vi "read-multiple-registers-rack.vi"(8 "error in":errorcluster, 9 "regs":u16[](array[numeric]), 10 "number of input registers":u16, 11 "TCP master in":refnum<class "Modbus Master.lvclass">) -> (0 "error out":errorcluster, 2 "Rack Cluster":T1, 3 "Modbus master out":refnum<class "Modbus Master.lvclass">)   [LabVIEW 2021]
uses:
  <vilib>/Modbus/master/Modbus Master.lvclass
  General Purpose/BMS.ctl
panel:
  in  "id":u16
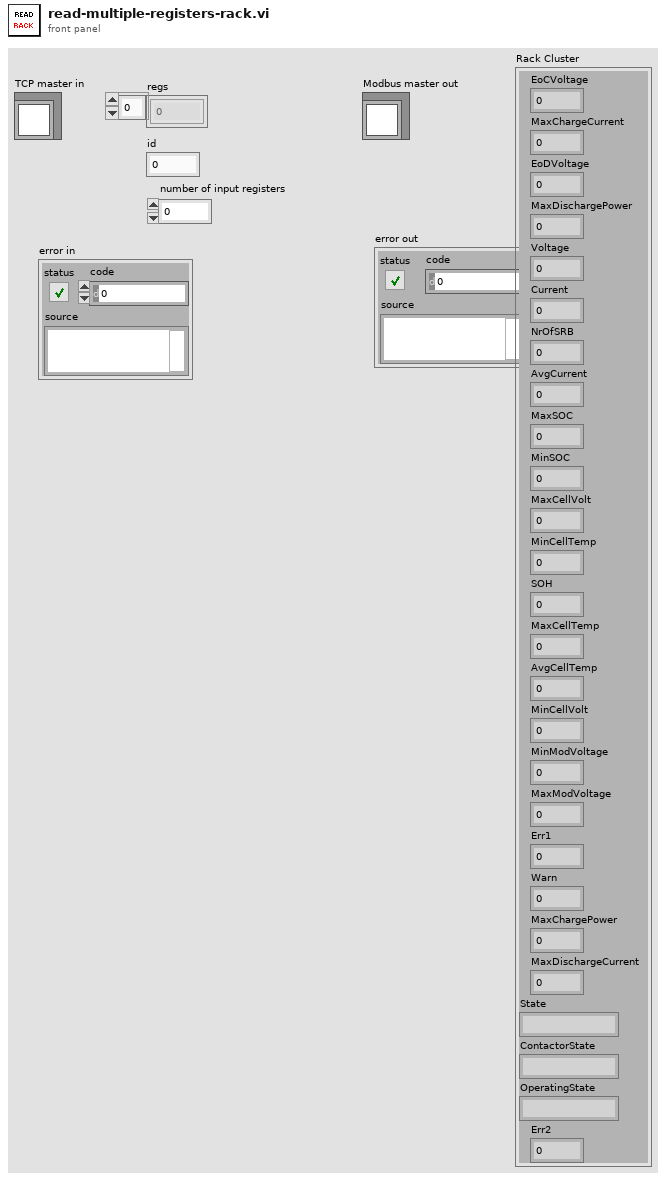
[diagram p1: front panel]
types:
  T1 = cluster{"EoCVoltage":dbl, "MaxChargeCurrent":dbl, "EoDVoltage":dbl, "MaxDischargePower":dbl, "Voltage":dbl, "Current":dbl, "NrOfSRB":u16, "AvgCurrent":dbl, "MaxSOC":u16, "MinSOC":u16, "MaxCellVolt":dbl, "MinCellTemp":dbl, "SOH":u16, "MaxCellTemp":dbl, "AvgCellTemp":dbl, "MinCellVolt":dbl, "MinModVoltage":dbl, "MaxModVoltage":dbl, "Err1":u16, "Warn":u16, "MaxChargePower":dbl, "MaxDischargeCurrent":dbl, "State":string, "ContactorState":string, "OperatingState":string, "Err2":u16}
  T2 = typedef "BMS.ctl" = cluster{"rack":cluster{"EoCVoltage":dbl, "MaxChargeCurrent":dbl, "EoDVoltage":dbl, "MaxDischargePower":dbl, "Voltage":dbl, "Current":dbl, "NrOfSRB":u16, "AvgCurrent":dbl, "MaxSOC":u16, "MinSOC":u16, "MaxCellVolt":dbl, "MinCellTemp":dbl, "SOH":u16, "MaxCellTemp":dbl, "AvgCellTemp":dbl, "MinCellVolt":dbl, "MinModVoltage":dbl, "MaxModVoltage":dbl, "Err1":u16, "Warn":u16, "MaxChargePower":dbl, "MaxDischargeCurrent":dbl, "State":string, "ContactorState":string, "OperatingState":string, "Err2":u16}[], "modules":cluster{"Voltage":dbl, "MaxCellTemp":dbl, "AirTempIn":dbl, "MinCellVoltage":u16, "AirTempOut":dbl, "MinSOC":u16, "MaxCellVoltage":u16, "Warn":u16, "SOH":u16, "MinCellTemp":dbl, "Err":u16, "Max SOC":u16}[]}
  T3 = cluster{"EoCVoltage":dbl, "MaxChargeCurrent":dbl, "EoDVoltage":dbl, "MaxDischargePower":dbl, "Voltage":dbl, "Current":dbl, "NrOfSRB":u16, "AvgCurrent":dbl, "MaxSOC":u16, "MinSOC":u16, "MaxCellVolt":dbl, "MinCellTemp":dbl, "SOH":u16, "MaxCellTemp":dbl, "AvgCellTemp":dbl, "MinCellVolt":dbl, "MinModVoltage":dbl, "MaxModVoltage":dbl, "Err1":u16, "Warn":u16, "MaxChargePower":dbl, "MaxDischargeCurrent":dbl, "State":string, "ContactorState":string, "OperatingState":string, "Err2":u16}[]
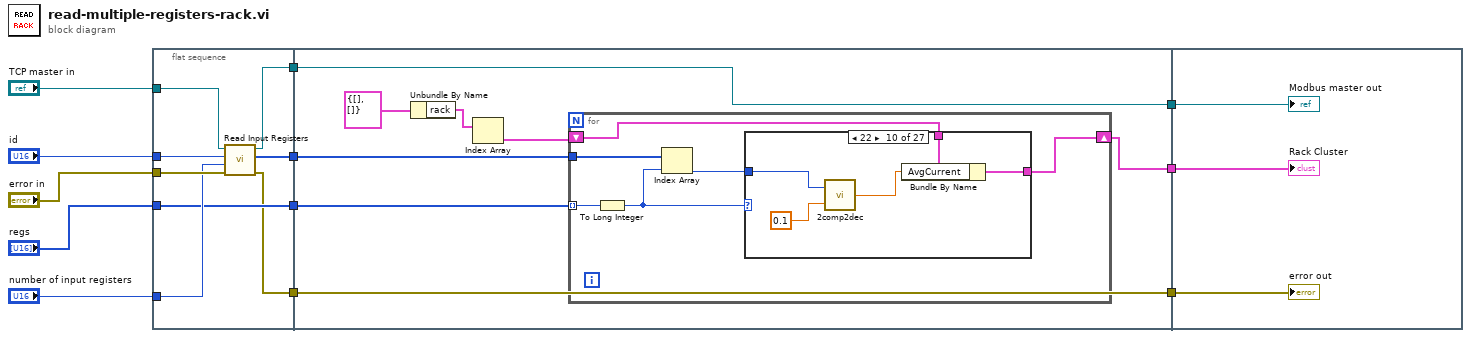
[diagram p0: block diagram]
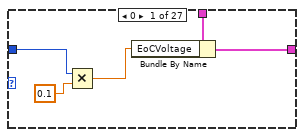
[diagram p2: hidden frame]
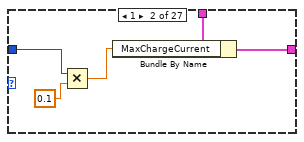
[diagram p3: hidden frame]
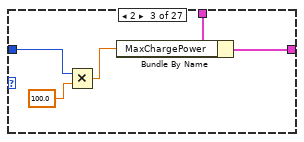
[diagram p4: hidden frame]
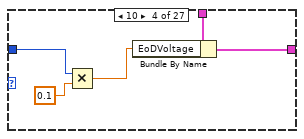
[diagram p5: hidden frame]
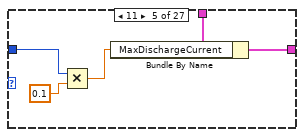
[diagram p6: hidden frame]
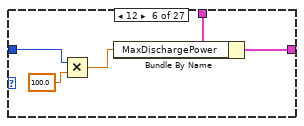
[diagram p7: hidden frame]
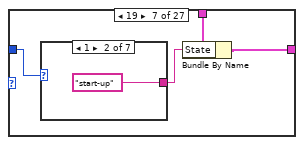
[diagram p8: hidden frame]
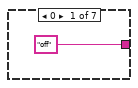
[diagram p9: hidden frame]
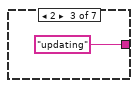
[diagram p10: hidden frame]
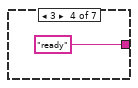
[diagram p11: hidden frame]
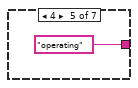
[diagram p12: hidden frame]
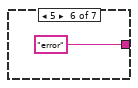
[diagram p13: hidden frame]
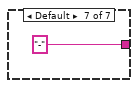
[diagram p14: hidden frame]
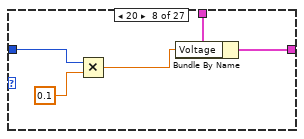
[diagram p15: hidden frame]
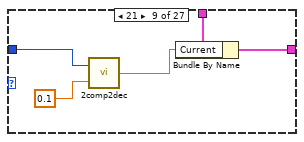
[diagram p16: hidden frame]
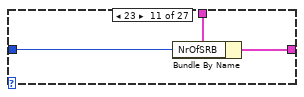
[diagram p17: hidden frame]
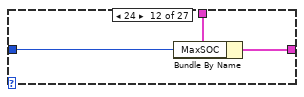
[diagram p18: hidden frame]
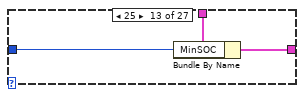
[diagram p19: hidden frame]
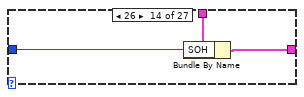
[diagram p20: hidden frame]
diagram:
  n1 = flat-sequence {
    tunnel: "TCP master in" -> [w20]
    tunnel: "id" -> [w19]
    tunnel: "error in" -> [w18]
    tunnel: "number of input registers" -> [w17]
    tunnel: [w16] -> w8
    tunnel: "regs" -> [w16]
    tunnel: [w15] -> w6
    tunnel: [w14] -> w3
    tunnel: [w13] -> w2
    tunnel: w8 -> [w28]
    tunnel: w6 -> [w27]
    tunnel: [w23] -> w5
    tunnel: [w22] -> w4
    tunnel: w3 -> [w22]
    tunnel: w2 -> [w21]
    tunnel: [w21] -> w1
    tunnel: w5 -> [w162]
    tunnel: w4 -> [w164]
    tunnel: w1 -> [w163]
    frame #0 {
      n2 = call-dynamic "Read Input Registers.vi"("error in (no error)"=w18, "number of input registers"=w17, "starting address"=w19, "Modbus master in"=w20) -> ("error out"=w13:errorcluster, "register values"=w15:u16[], "Modbus master out"=w14:refnum<class "Modbus Master.lvclass">)  [unwired: 5 in]
    }
    frame #1 {
      n3 = Unbundle By Name(T2 {"rack"=[], "modules"=[]} ("BMS")) -> ("rack"=w25:T3)
      n4 = Index Array(array=w25) -> (element=w24:T1)  [unwired: 1 in]
      n5 = for {
        tunnel: w28 -> [w34] mode=indexing
        tunnel: w27 -> [w33]
        shift-right: [w29] -> w23
        shift-left: w24 -> [w30]
        n6 = To Long Integer(number=w34) -> (32bit integer=w31:i32)
        n7 = Index Array(array=w33, index=w31) -> (element=w32:u16)
        n8 = case shown="22" w31 {
          tunnel: w32 -> [w37 w42 w46 w52 w57 w61 w66 w77 w83 w87 w91 w94 w97 w100 w104 w109 w117 w122 w127 w131 w134 w139 w145 w152 w155 w158 _]
          tunnel: w30 -> [w39 w44 w49 w54 w59 w64 w68 w80 w85 w90 w93 w96 w99 w102 w107 w111 w120 w125 w129 w133 w138 w143 w147 w154 w157 w160 w161]
          tunnel: [w38 w43 w48 w53 w58 w63 w67 w79 w84 w89 w92 w95 w98 w101 w106 w110 w119 w124 w128 w132 w137 w142 w146 w153 w156 w159 w161] -> w29
          frame 0 {
            n9 = Multiply(x=w37, y=0.1) -> (x*y=w36:dbl)
            n10 = Bundle By Name(cluster=w39, "EoCVoltage"=w36) -> (w38:T1)
          }
          frame 1 {
            n11 = Multiply(x=w42, y=0.1) -> (x*y=w40:dbl)
            n12 = Bundle By Name(cluster=w44, "MaxChargeCurrent"=w40) -> (w43:T1)
          }
          frame 2 {
            n13 = Multiply(x=w46, y=100.0) -> (x*y=w45:dbl)
            n14 = Bundle By Name(cluster=w49, "MaxChargePower"=w45) -> (w48:T1)
          }
          frame 10 {
            n15 = Multiply(x=w52, y=0.1 ("x")) -> (x*y=w50:dbl)
            n16 = Bundle By Name(cluster=w54, "EoDVoltage"=w50) -> (w53:T1)
          }
          frame 11 {
            n17 = Multiply(x=w57, y=0.1) -> (x*y=w55:dbl)
            n18 = Bundle By Name(cluster=w59, "MaxDischargeCurrent"=w55) -> (w58:T1)
          }
          frame 12 {
            n19 = Multiply(x=w61, y=100.0) -> (x*y=w60:dbl)
            n20 = Bundle By Name(cluster=w64, "MaxDischargePower"=w60) -> (w63:T1)
          }
          frame 19 {
            n21 = case shown="1" w66 {
              tunnel: ["off" "start-up" "updating" "ready" "operating" "error" "-"] -> w65
              frame 0 {
              }
              frame 1 {
              }
              frame 2 {
              }
              frame 3 {
              }
              frame 4 {
              }
              frame 5 {
              }
              frame Default {
              }
            }
            n22 = Bundle By Name(cluster=w68, "State"=w65) -> (w67:T1)
          }
          frame 20 {
            n23 = Multiply(x=w77, y=0.1) -> (x*y=w76:dbl)
            n24 = Bundle By Name(cluster=w80, "Voltage"=w76) -> (w79:T1)
          }
          frame 21 {
            n25 = call "2comp2dec.vi"("factor"=0.1, "two' complement"=w83) -> ("decimal"=w82:dbl)  [unwired: 1 in]
            n26 = Bundle By Name(cluster=w85, "Current"=w82) -> (w84:T1)
          }
          frame 22 {
            n27 = call "2comp2dec.vi"("factor"=0.1, "two' complement"=w87) -> ("decimal"=w86:dbl)  [unwired: 1 in]
            n28 = Bundle By Name(cluster=w90, "AvgCurrent"=w86) -> (w89:T1)
          }
          frame 23 {
            n29 = Bundle By Name(cluster=w93, "NrOfSRB"=w91) -> (w92:T1)
          }
          frame 24 {
            n30 = Bundle By Name(cluster=w96, "MaxSOC"=w94) -> (w95:T1)
          }
          frame 25 {
            n31 = Bundle By Name(cluster=w99, "MinSOC"=w97) -> (w98:T1)
          }
          frame 26 {
            n32 = Bundle By Name(cluster=w102, "SOH"=w100) -> (w101:T1)
          }
          frame 31 {
            n33 = call "2comp2dec.vi"("factor"=1.0, "two' complement"=w104) -> ("decimal"=w103:dbl)  [unwired: 1 in]
            n34 = Bundle By Name(cluster=w107, "AvgCellTemp"=w103) -> (w106:T1)
          }
          frame 33 {
            n35 = case shown="2" w109 {
              tunnel: ["open" "pre-charge" "closed" "-"] -> w108
              frame 0 {
              }
              frame 1 {
              }
              frame 2 {
              }
              frame Default {
              }
            }
            n36 = Bundle By Name(cluster=w111, "ContactorState"=w108) -> (w110:T1)
          }
          frame 34 {
            n37 = Multiply(x=w117, y=0.001) -> (x*y=w116:dbl)
            n38 = Bundle By Name(cluster=w120, "MinCellVolt"=w116) -> (w119:T1)
          }
          frame 35 {
            n39 = Multiply(x=w122, y=0.001) -> (x*y=w121:dbl)
            n40 = Bundle By Name(cluster=w125, "MaxCellVolt"=w121) -> (w124:T1)
          }
          frame 36 {
            n41 = call "2comp2dec.vi"("two' complement"=w127) -> ("decimal"=w126:dbl)  [unwired: 2 in]
            n42 = Bundle By Name(cluster=w129, "MinCellTemp"=w126) -> (w128:T1)
          }
          frame 37 {
            n43 = call "2comp2dec.vi"("two' complement"=w131) -> ("decimal"=w130:dbl)  [unwired: 2 in]
            n44 = Bundle By Name(cluster=w133, "MaxCellTemp"=w130) -> (w132:T1)
          }
          frame 38 {
            n45 = Multiply(x=w134, y=0.01) -> (x*y=w136:dbl)
            n46 = Bundle By Name(cluster=w138, "MinModVoltage"=w136) -> (w137:T1)
          }
          frame 39 {
            n47 = Multiply(x=w139, y=0.01) -> (x*y=w141:dbl)
            n48 = Bundle By Name(cluster=w143, "MaxModVoltage"=w141) -> (w142:T1)
          }
          frame 52 {
            n49 = case shown="Default" w145 {
              tunnel: ["discharge" "charge" "idle" "-"] -> w144
              frame 1 {
              }
              frame 2 {
              }
              frame 3 {
              }
              frame Default {
              }
            }
            n50 = Bundle By Name(cluster=w147, "OperatingState"=w144) -> (w146:T1)
          }
          frame 70 {
            n51 = Bundle By Name(cluster=w154, "Err1"=w152) -> (w153:T1)
          }
          frame 71 {
            n52 = Bundle By Name(cluster=w157, "Err2"=w155) -> (w156:T1)
          }
          frame 74 {
            n53 = Bundle By Name(cluster=w160, "Warn"=w158) -> (w159:T1)
          }
          frame Default {
          }
        }
      }
    }
    frame #2 {
      "error out" <- w163
      "Modbus master out" <- w164
      "Rack Cluster" <- w162
    }
  }
